vi "runReady.vi"(4 "FullRun? in":bool, 6 "Fault?":bool, 7 "Time in":dbl, 8 "error in":errorcluster, 9 "Actuators in":T2, 10 "State in":T1, 11 "SystemsCheck in":refnum<class "SystemsCheck.lvclass">) -> (0 "error out":errorcluster, 1 "Actuators out":T2, 2 "State out":T1, 3 "SystemsCheck out":refnum<class "SystemsCheck.lvclass">, 5 "FullRun? out":bool)   [LabVIEW 2018, in "ControlLibrary.lvlib" / "SystemsCheck.lvclass"]
uses:
  SystemsCheck.lvclass
  TypeDef_DigitalOuts.ctl
  TypeDef_ControlState.ctl
  RunTypeList.ctl
  RunTypeClass/RunType.lvclass
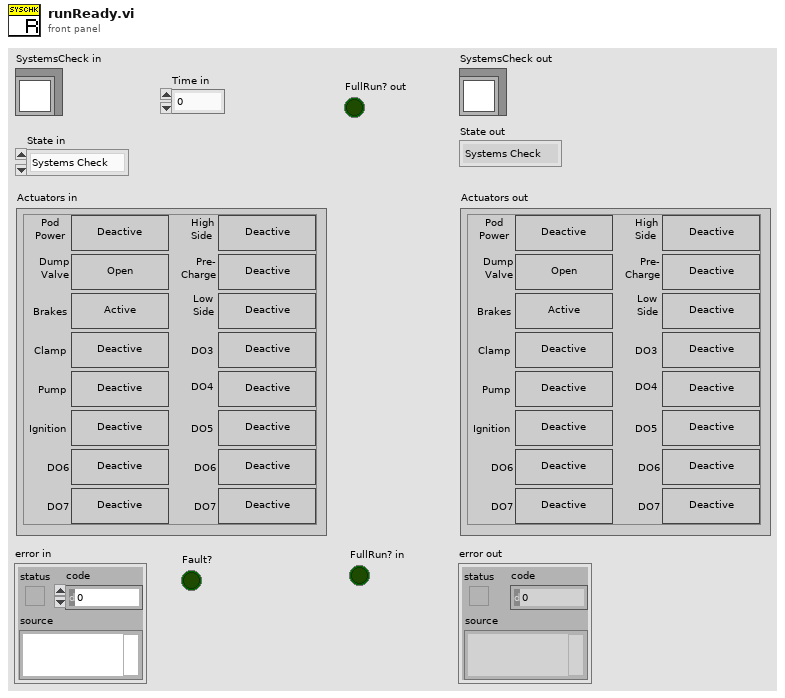
[diagram p1: front panel]
types:
  T1 = typedef "TypeDef_ControlState.ctl" = enum16{"Systems Check", "Idle", "Ready", "Pushing", "Coast", "Braking", "Fault", "Shutdown", "Service", "Precharge", "Blank"}
  T2 = typedef "TypeDef_DigitalOuts.ctl" = cluster{"Pod Power":bool, "Dump Valve":bool, "Brakes":bool, "Clamp":bool, "Pump":bool, "Ignition":bool, "DO6":bool, "DO7":bool, "HighSide":bool, "Precharge":bool, "LowSide":bool, "DO3":bool, "DO4":bool, "DO5":bool, "DO62":bool, "DO72":bool}
  T3 = typedef "RunTypeList.ctl" = enum16{"Full Run", "Systems Check", "Service"}
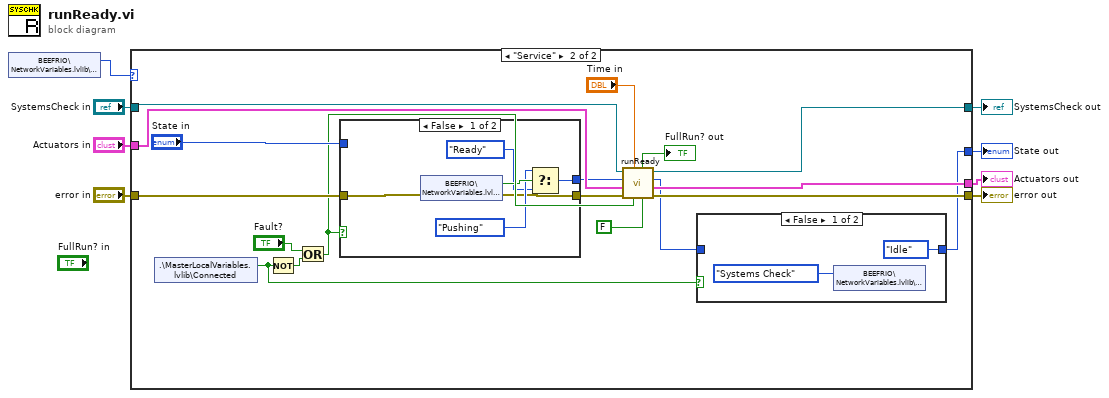
[diagram p0: block diagram]
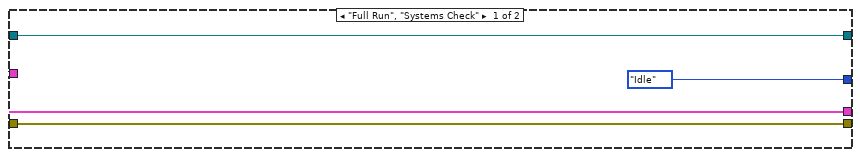
[diagram p2: hidden frame]
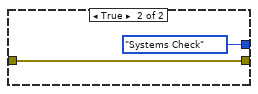
[diagram p4: hidden frame]
diagram:
  n1 = shared-variable "BEEFRIO\\NetworkVariables.lvlib\\RunType"() -> (w1:T3)  [unwired: 1 in, 1 out]
  n2 = case shown="\"Service\"" w1 {
    tunnel: [w10 w30] -> w8
    tunnel: [w11 w29] -> w7
    tunnel: [TypeDef_ControlState."Idle" ("State out") w13] -> w6
    tunnel: [w12 w28] -> w5
    tunnel: "Actuators in" -> [w11 w25]
    tunnel: "SystemsCheck in" -> [w12 w24]
    tunnel: "error in" -> [w10 w19]
    frame "Full Run", "Systems Check" {
    }
    frame "Service" {
      n3 = shared-variable ".\\MasterLocalVariables.lvlib\\Connected"() -> (w15:bool)  [unwired: 1 in, 1 out]
      n4 = Not(x=w15) -> (.not. x?=w16:bool)
      n5 = Or(x="Fault?", y=w16) -> (x .or. y?=w18:bool)
      n6 = case shown="False" w18 {
        tunnel: "State in" -> [_ _]
        tunnel: [w38 TypeDef_ControlState."Systems Check" ("State in")] -> w22
        tunnel: w19 -> [w35 w40]
        tunnel: [w34 w40] -> w21
        frame False {
          n7 = shared-variable "BEEFRIO\\NetworkVariables.lvlib\\Service"(error in=w35) -> (w39:bool, error out=w34:errorcluster)
          n8 = Select(t=TypeDef_ControlState."Pushing" ("State in"), s=w39, f=TypeDef_ControlState."Ready" ("State in")) -> (s? t:f=w38:T1)
        }
        frame True {
        }
      }
      n9 = call-parent "runReady.vi"("FullRun? in"=FALSE, "Fault?"=w18, "Time in"="Time in", "error in (no error)"=w21, "Actuators in"=w25, "State in"=w22, "RunType in"=w24) -> ("error out"=w30:errorcluster, "Actuators out"=w29:T2, "State out"=w14:T1, "RunType out"=w28:refnum<class "SystemsCheck.lvclass">, "FullRun? out"=→"FullRun? out":bool)
      n10 = case shown="False" w15 {
        tunnel: w14 -> [_ w33]
        tunnel: [TypeDef_ControlState."Idle" ("State out") w33] -> w13
        frame False {
          n11 = shared-variable "BEEFRIO\\NetworkVariables.lvlib\\RunType"(RunTypeList."Systems Check" ("RunType")) -> ()  [unwired: 1 in, 1 out]
        }
        frame True {
        }
      }
    }
  }
  "error out" <- w8
  "SystemsCheck out" <- w5
  "State out" <- w6
  "Actuators out" <- w7
